vi "Do.vi"(8 "error in":errorcluster, 10 "Actor in":refnum<class "Actor.lvclass">, 11 "Change Filter State":refnum<class "Change Filter State.lvclass">) -> (0 "error out":errorcluster, 2 "Actor out":refnum<class "Actor.lvclass">)   [LabVIEW 2014, in "ePAS Library.lvlib" / "Change Filter State.lvclass"]
doc: "(<B>Filename</B>: Actor Framework.lvlib:Message.lvclass:Do.vi)\n\nDefines what a message does when it is received by an actor. Generally, a message instructs an actor to invoke one of its methods. By default, this method does nothing. A child class must override it to define behavior. Create a child class by using the Actor Framework Message Maker dialog box."
uses:
  Change Filter State.lvclass
  <vilib>/ActorFramework/Actor/Actor.lvclass
  Change Filter State.lvclass/Change Filter State.ctl
  Instr Actor/Instr Actor.lvclass
  Commands/Update Filter State/Update Filter State CMD.lvclass
  Commands/Update Filter State/Update Filter State CMD.lvclass/Update Filter State CMD.ctl
  Commands/Update Filter State/Write State.vi
  Instr Actor/Accessors/Read CMD.vi
  reusable/Command/Command.lvclass
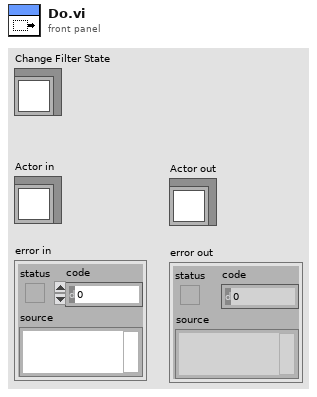
[diagram p1: front panel]
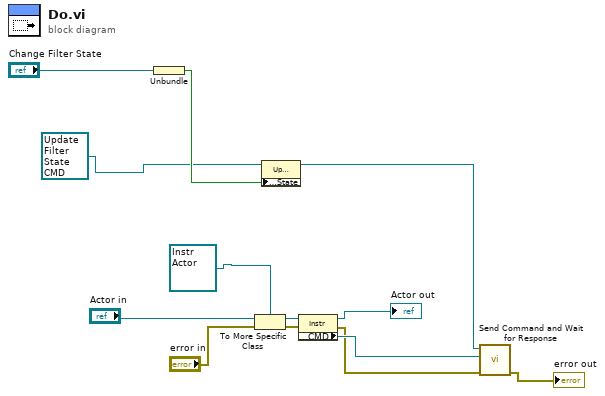
[diagram p0: block diagram]
diagram:
  n1 = Unbundle("Change Filter State") -> (w3:bool)
  n2 = To More Specific Class(target class=refnum<class "Instr Actor.lvclass"> refnum ("Instrument Lib:Instr"), reference="Actor in", error in="error in") -> (specific class reference=w13:refnum<class "Instr Actor.lvclass">, error out=w12:errorcluster)
  n3 = property class="Update Filter State CMD.lvclass"(reference=refnum<class "Update Filter State CMD.lvclass"> refnum ("ePAS Library.lvlib:Update Filter State CMD.lvclass"), "Accessors:State"=w3) -> (reference out=w2:refnum<class "Update Filter State CMD.lvclass">)  [unwired: 1 in, 1 out]
  n4 = property class="Instr"(reference=w13, error in=w12) -> (reference out=→"Actor out":refnum<class "Instr Actor.lvclass">, error out=w10:errorcluster, "Accessors:CMD"=w11:refnum<queue>)
  n5 = call "Send Command and Wait for Response.vi"("error in"=w10, "cmd queue"=w11, "CMD in"=w2) -> ("error out"=→"error out":errorcluster)  [unwired: 6 in, 2 out]
